vi "postiontesting.vi"() -> ()   [LabVIEW 2017]
uses:
  <vilib>/Simulation/Scripting/Companion Diagram/SimConfigNode/SimParams.ctl
  <vilib>/Simulation/Scripting/Companion Diagram/SimConfigNode/_simSolvers.ctl
  <vilib>/Simulation/Implementation/Shared/SIMSCR Execution Mode.ctl
  <vilib>/Simulation/Param Hierarchy/Typedefs/SIMPH Param Control Actions.ctl
  <vilib>/Simulation/Implementation/Shared/NILVSim_ParamChanged.vi
  <vilib>/Simulation/Implementation/Shared/NILVSIM_BeginStep.vi
  <vilib>/Simulation/Implementation/Shared/NILVSim_Manager.vi
  <vilib>/Utility/error.llb/Clear Errors.vi
  <vilib>/Simulation/Implementation/Shared/NILVSim_FinalizeModel.vi
  <vilib>/DAQmx/read.llb/DAQmx Read (Counter DBL 1Chan 1Samp).vi
  <vilib>/DAQmx/read.llb/DAQmx Read (Digital Bool 1Line 1Point).vi
  <vilib>/DAQmx/write.llb/DAQmx Write (Analog DBL 1Chan 1Samp).vi
  <vilib>/DAQmx/create/channels.llb/DAQmx Create Channel (AO-Voltage-Basic).vi
  <vilib>/DAQmx/create/channels.llb/DAQmx Create Channel (DI-Digital Input).vi
  <vilib>/DAQmx/create/channels.llb/DAQmx Create Channel (CI-Count Edges).vi
  <vilib>/Simulation/Implementation/Shared/SIM Unbundle Sim Info.vi
  <vilib>/Simulation/Implementation/Shared/NILVSim_Initialize.vi
  <vilib>/Simulation/Utility/Implementation/NILVSim Get Time and IsAcceptedStep.vi
  <vilib>/Simulation/Implementation/Shared/SIMSH Read Queue.vi
  <vilib>/Simulation/Implementation/Shared/NILVSim_GetModelError.vi
  <vilib>/Simulation/Implementation/Shared/SIM Bundle Sim Info.vi
  <vilib>/DAQmx/miscellaneous.llb/DAQmx Fill In Error Info.vi
  <vilib>/Simulation/Implementation/XNodeFramework/SimXNode/SimX.xnode
  <vilib>/Simulation/Model Libraries/PID/SIM PID (Parallel).vi
  <vilib>/Simulation/Model Libraries/PID/SIM PID.vi
  <vilib>/Simulation/Scripting/Companion Diagram/SimConfigNode/SimDog.xnode
  <vilib>/Simulation/Model Libraries/PID/SIM PID (Academic).vi
  <vilib>/Simulation/Implementation/Shared/NI_SIM_Implementation.lvlib
panel:
  in  "Draw rectangle":bool
  in  "Draw circle":bool
  out "In drawing mode":bool
  in  "Right-Down":bool
  in  "Left-Up":bool
  in  "Left-Down":bool
  in  "Right-Up":bool
  in  "right":bool
  in  "left":bool
  in  "motor 2":dbl(slide)=1.5 scale=-10.0..10.0
  in  "down":bool
  in  "up":bool
  in  "Length 2":dbl
  in  "Length 1":dbl
  in  "Motor 2 encoder":tag="Dev9/ao0"
  out "Pulses M2":dbl format="%.2f"
  in  "Motor 1 encoder":tag="Dev9/ao0"
  out "Pulses M1":dbl format="%.2f"
  out "Right":bool
  out "Bottom":bool
  out "Left":bool
  out "Top":bool
  in  "Switch 4/Line 3":tag
  in  "Switch 3/Line 2":tag
  in  "Switch 2/Line 1":tag
  in  "Switch 1/Line 0":tag
  in  "Motor stop":bool
  in  "Motor 1":tag="Dev9/ao0"
  in  "max Voltage":dbl
  in  "Min Voltage":dbl
  in  "Motor 2":tag="Dev9/ao0"
  in  "motor 1":dbl(slide)=1.5 scale=-10.0..10.0
  in  "stop":bool
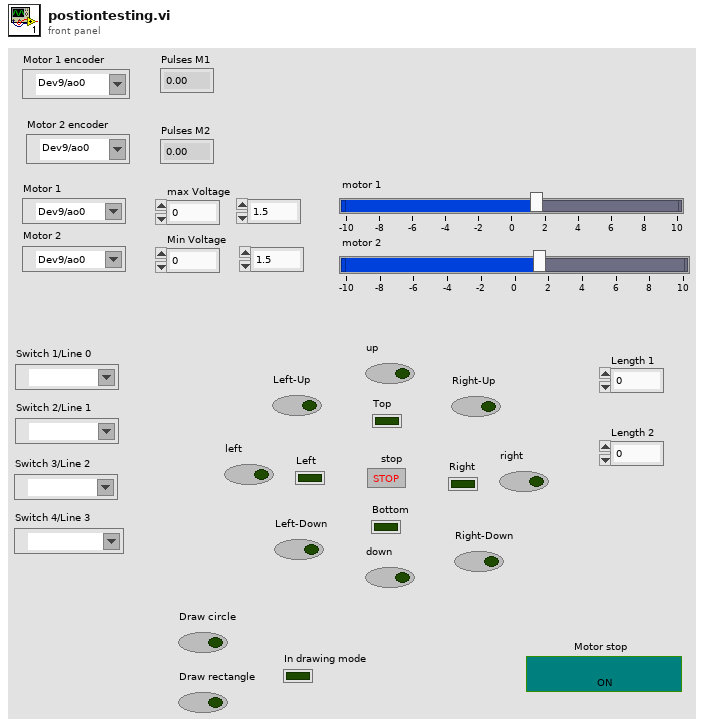
[diagram p1: front panel]
types:
  T1 = enum16{"Simulate to Completion", "Single Time-Step Simulation (Fixed Step Only)"}
  T2 = typedef "SIMSCR Execution Mode.ctl" = enum16{"Simulate to Completion", "Single Time-Step Simulation (Fixed Step Only)"}
  T3 = typedef "SIMPH Param Control Actions.ctl" = enum16{"get params", "set params"}
  T4 = cluster{"SIMSH Sim Time":dbl, "SIM PID Derivative Gain.vi":cluster{"output":dbl}, "SIM PID Derivative Gain.vi - SIMSH":cluster{"SIMSH Sim Time":dbl, "t 3":dbl, "Select 2":cluster{"s? t:f":dbl}, "Equal?":cluster{"x = y?":bool}, "Or":cluster{"x .or. y?":bool}, "Equal To 0?":cluster{"x = 0?":bool}}, "High Frequency [s] (Tf)":dbl, "Gain":cluster{"output":dbl}, "Summation":cluster{"Result":dbl}, "Integral Gain - series.vi":cluster{"output":dbl}, "Integral Gain - series.vi - SIMSH":cluster{"SIMSH Sim Time":dbl, "Select 2":cluster{"s? t:f":dbl}, "integral in gain?":bool, "Integrator":cluster{"output y(t)":dbl}, "Gain 2":cluster{"output":dbl}, "Select":cluster{"s? t:f":dbl}, "Equal To 0?":cluster{"x = 0?":bool}, "Reciprocal":cluster{"1/x":dbl}}}
  T5 = typedef "SimParams.ctl" = cluster{"Initial Time (s)":dbl, "Final Time (s)":dbl, "Step Size (s)":dbl, "ODE Solver":T6, "Minimum Step Size (s)":dbl, "Maximum Step Size (s)":dbl, "Relative Tolerance":dbl, "Absolute Tolerance":dbl, "Software Timing":bool, "Initial Step Size (s)":dbl, "Automatic Fixed Step Size?":bool, "Automatic Discrete Step Size?":bool, "Discrete Step Size (s)":dbl, "Calculate using Time Step":bool, "Solver Wired?":bool, "Prev.Frm.Expected End":u64, "Prev.Frm.Actual End":u64, "Prev.Frm.Finished Late?":bool, "Prev.Iter.Expected End":u64, "Prev.Iter.Actual End":u64, "Prev.Iter.Finished Late?":bool, "Expected Iteration Start":u64, "Actual Iteration Start":u64, "Expected Frame Start":u64, "Actual Frame Start":u64, "Source Name":string, "Name":string, "Period":i64, "Deadline":i64, "Offset":i64, "Start":i64, "Priority":i32, "Timeout":i32, "Processor":i32, "Mode":enum32{"No Change", "Process missed periods, maintain original phase", "Discard missed periods, maintain original phase", "Process missed periods, ignore original phase", "Discard missed periods, ignore original phase"}, "Wakeup reason":enum32{"Normal", "Aborted", "Asynchronous wakeup", "Timing source error", "Timed loop error", "Timeout"}, "Error":errorcluster, "Source Type":string, "Secondary Source Type":string, "Global End Time":u64, "Global Start Time":u64, "Full Solver Reset":bool, "Execution Mode":T2, "Nan/Inf Check":bool, "Custom Solver Library":string, "Solver Is Variable":bool, "custom solver name":string, "Signal Collection Decimation":u32}
  T6 = typedef "_simSolvers.ctl" = enum16{"Runge-Kutta 1 (Euler)", "Runge-Kutta 2", "Runge-Kutta 3", "Runge-Kutta 4", "Runge-Kutta 23 (variable)", "Runge-Kutta 45 (variable)", "BDF (variable)", "Adams-Moulton (variable)", "Rosenbrock (variable)", "Discrete States Only", "SDIRK 4 (variable)", "Radau 5 (variable)", "Radau 9 (variable)", "Radau 13 (variable)", "Radau [Variable Order] (variable)", "Gear's Method (variable)", "Linearizer", "State Query", "Trim Eval", "Custom Solver"}
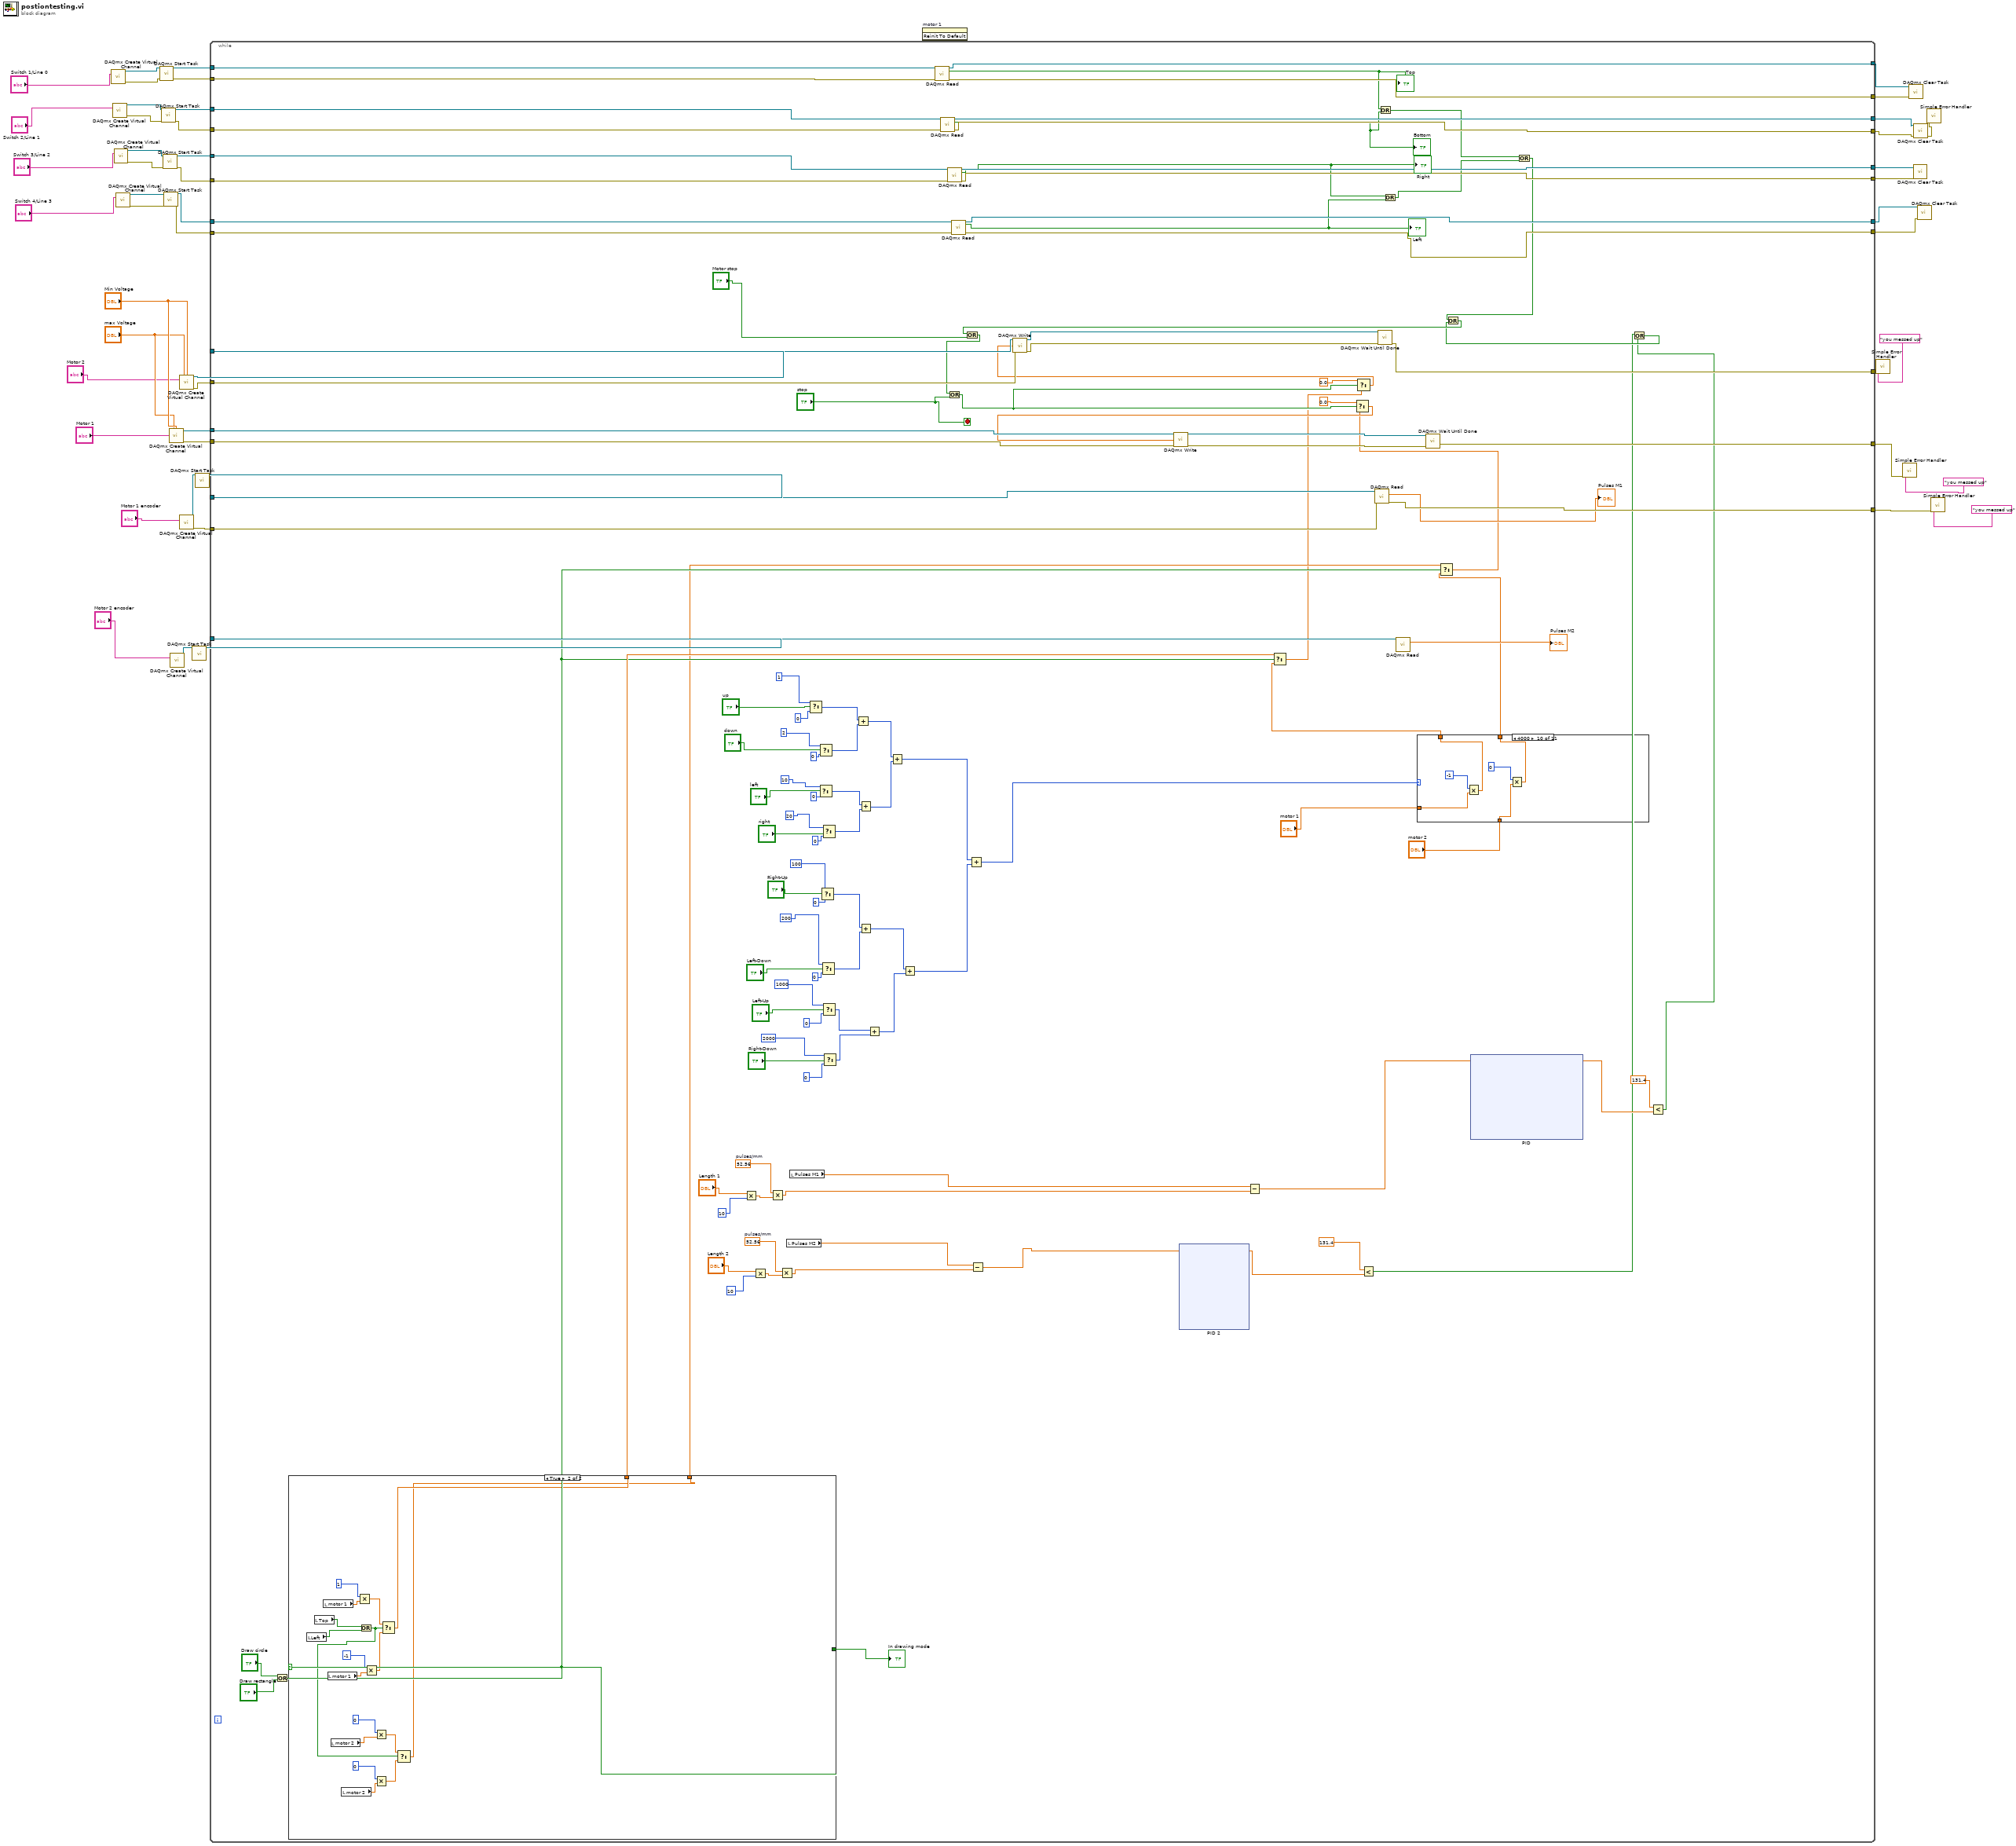
[diagram p0: block diagram]
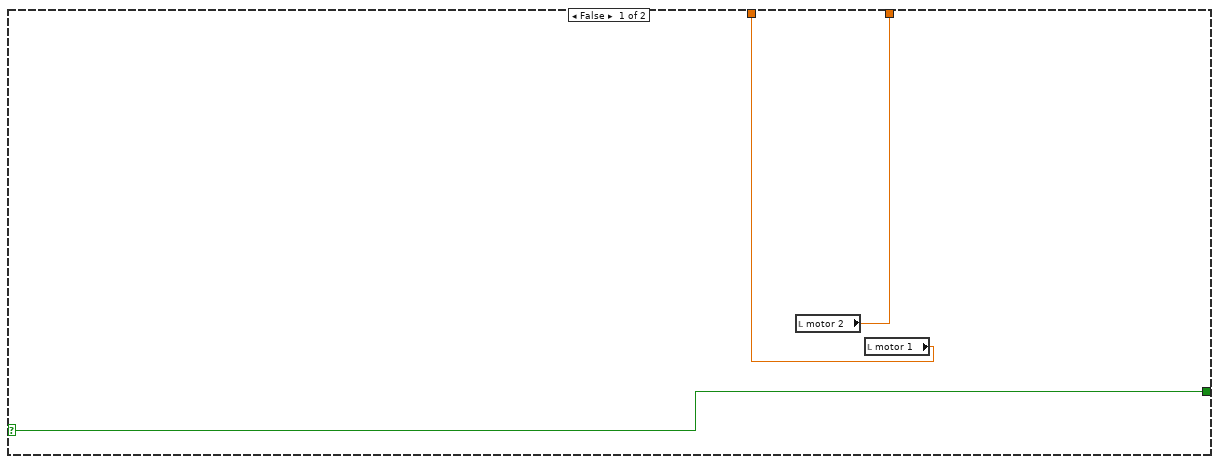
[diagram p2: hidden frame]
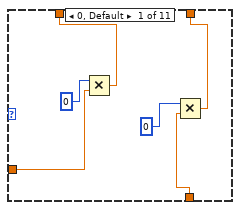
[diagram p3: hidden frame]
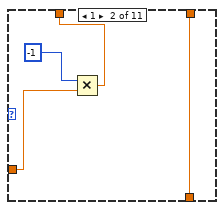
[diagram p4: hidden frame]
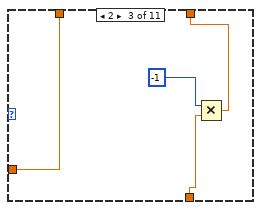
[diagram p5: hidden frame]
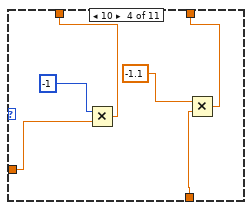
[diagram p6: hidden frame]
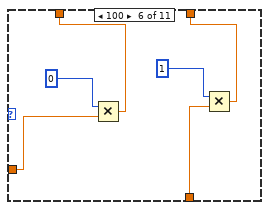
[diagram p8: hidden frame]
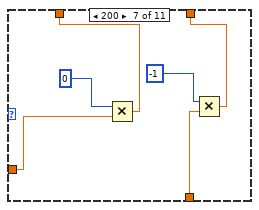
[diagram p9: hidden frame]
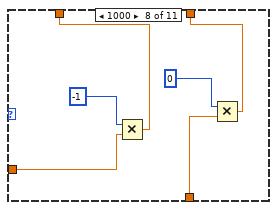
[diagram p10: hidden frame]
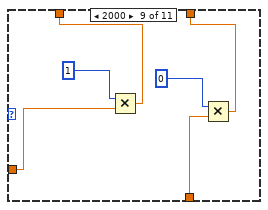
[diagram p11: hidden frame]
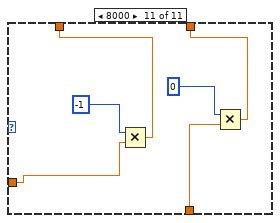
[diagram p12: hidden frame]
diagram:
  n1 = call-poly <vilib>:"DAQmx Create Virtual Channel.vi"("lines"="Switch 1/Line 0") -> ("task out"=w36:refnum<k21>, "error out"=w32:errorcluster)  [unwired: 13 in]
  n2 = call-poly <vilib>:"DAQmx Create Virtual Channel.vi"("lines"="Switch 2/Line 1") -> ("task out"=w35:refnum<k21>, "error out"=w31:errorcluster)  [unwired: 13 in]
  n3 = call-poly <vilib>:"DAQmx Create Virtual Channel.vi"("lines"="Switch 3/Line 2") -> ("task out"=w34:refnum<k21>, "error out"=w30:errorcluster)  [unwired: 13 in]
  n4 = call-poly <vilib>:"DAQmx Create Virtual Channel.vi"("lines"="Switch 4/Line 3") -> ("task out"=w33:refnum<k21>, "error out"=w29:errorcluster)  [unwired: 13 in]
  n5 = call <vilib>:"DAQmx Start Task.vi"("task/channels in"=w36, "error in"=w32) -> ("task out"=w28:refnum<k21>, "error out"=w26:errorcluster)  [unwired: 12 in]
  n6 = call <vilib>:"DAQmx Start Task.vi"("task/channels in"=w35, "error in"=w31) -> ("task out"=w24:refnum<k21>, "error out"=w21:errorcluster)  [unwired: 12 in]
  n7 = call <vilib>:"DAQmx Start Task.vi"("task/channels in"=w34, "error in"=w30) -> ("task out"=w23:refnum<k21>, "error out"=w20:errorcluster)  [unwired: 12 in]
  n8 = call <vilib>:"DAQmx Start Task.vi"("task/channels in"=w33, "error in"=w29) -> ("task out"=w22:refnum<k21>, "error out"=w19:errorcluster)  [unwired: 12 in]
  n9 = call-poly <vilib>:"DAQmx Create Virtual Channel.vi"("maximum value"="max Voltage", "minimum value"="Min Voltage", "physical channels"="Motor 1") -> ("task out"=w46:refnum<k21>, "error out"=w42:errorcluster)  [unwired: 11 in]
  n10 = call-poly <vilib>:"DAQmx Create Virtual Channel.vi"("counter"="Motor 2 encoder") -> ("task out"=w4:refnum<k21>)  [unwired: 13 in, 1 out]
  n11 = call-poly <vilib>:"DAQmx Create Virtual Channel.vi"("maximum value"="max Voltage", "minimum value"="Min Voltage", "physical channels"="Motor 2") -> ("task out"=w49:refnum<k21>, "error out"=w41:errorcluster)  [unwired: 11 in]
  n12 = call-poly <vilib>:"DAQmx Create Virtual Channel.vi"("counter"="Motor 1 encoder") -> ("task out"=w6:refnum<k21>, "error out"=w7:errorcluster)  [unwired: 13 in]
  n13 = call <vilib>:"DAQmx Start Task.vi"("task/channels in"=w4) -> ("task out"=w3:refnum<k21>)  [unwired: 13 in, 1 out]
  n14 = call <vilib>:"DAQmx Start Task.vi"("task/channels in"=w6) -> ("task out"=w5:refnum<k21>)  [unwired: 13 in, 1 out]
  n15 = while {
    tunnel: w49 -> [w170]
    tunnel: [w167] -> w48
    tunnel: w46 -> [w164]
    tunnel: [w163] -> w45
    tunnel: w42 -> [w161]
    tunnel: w41 -> [w160]
    tunnel: w28 -> [w154]
    tunnel: [w153] -> w27
    tunnel: w26 -> [w152]
    tunnel: [w151] -> w25
    tunnel: w24 -> [w150]
    tunnel: w23 -> [w149]
    tunnel: w22 -> [w148]
    tunnel: w21 -> [w147]
    tunnel: w20 -> [w146]
    tunnel: w19 -> [w145]
    tunnel: [w144] -> w18
    tunnel: [w143] -> w17
    tunnel: [w142] -> w16
    tunnel: [w141] -> w15
    tunnel: [w140] -> w14
    tunnel: [w139] -> w13
    tunnel: [w138] -> w10
    tunnel: w5 -> [w137]
    tunnel: w7 -> [w136]
    tunnel: w3 -> [w127]
    stop <- "stop" stop-if-true
    w117 = 52.56  # pulses/mm
    w122 = 52.56  # pulses/mm
    n16 = Or(x="Draw circle", y="Draw rectangle") -> (x .or. y?=w56:bool)
    n17 = case shown="True" w56 {
      selector: w56 -> [w173 w191]
      tunnel: [w173 w191] -> w60
      tunnel: [w172 w176] -> w57
      tunnel: [w171 w175] -> w55
      frame False {
        n18 = local read "motor 2"() -> (w171:dbl)
        n19 = local read "motor 1"() -> (w172:dbl)
      }
      frame True {
        n20 = local read "Left"() -> (w174:bool)
        n21 = local read "Top"() -> (w190:bool)
        n22 = local read "motor 1"() -> (w187:dbl)
        n23 = local read "motor 1"() -> (w181:dbl)
        n24 = local read "motor 2"() -> (w185:dbl)
        n25 = local read "motor 2"() -> (w178:dbl)
        n26 = Multiply(x=1, y=w187) -> (x*y=w186:dbl)
        n27 = Or(x=w190, y=w174) -> (x .or. y?=w183:bool)
        n28 = Multiply(x=-1, y=w181) -> (x*y=w180:dbl)
        n29 = Multiply(x=0, y=w185) -> (x*y=w184:dbl)
        n30 = Multiply(x=0, y=w178) -> (x*y=w177:dbl)
        n31 = Select(t=w186, s=w183, f=w180) -> (s? t:f=w176:dbl)
        n32 = Select(t=w184, s=w183, f=w177) -> (s? t:f=w175:dbl)
      }
    }
    "In drawing mode" <- w60
    n33 = Multiply(x="Length 1", y=10) -> (x*y=w121:dbl)
    n34 = Multiply(x="Length 2", y=10) -> (x*y=w120:dbl)
    n35 = Multiply(x=w122, y=w121) -> (x*y=w110:dbl)
    n36 = Multiply(x=w117, y=w120) -> (x*y=w104:dbl)
    n37 = local read "Pulses M2"() -> (w105:dbl)
    n38 = local read "Pulses M1"() -> (w111:dbl)
    n39 = Select(t=1, s="up", f=0) -> (s? t:f=w84:i32)
    n40 = Select(t=10, s="left", f=0) -> (s? t:f=w82:i32)
    n41 = Select(t=2, s="down", f=0) -> (s? t:f=w83:i32)
    n42 = Select(t=100, s="Right-Up", f=0) -> (s? t:f=w80:i32)
    n43 = Select(t=200, s="Left-Down", f=0) -> (s? t:f=w79:i32)
    n44 = Select(t=20, s="right", f=0) -> (s? t:f=w81:i32)
    n45 = Select(t=1000, s="Left-Up", f=0) -> (s? t:f=w78:i32)
    n46 = Select(t=2000, s="Right-Down", f=0) -> (s? t:f=w64:i32)
    n47 = Add(x=w84, y=w83) -> (x+y=w77:i32)
    n48 = Add(x=w82, y=w81) -> (x+y=w76:i32)
    n49 = Add(x=w80, y=w79) -> (x+y=w75:i32)
    n50 = Add(x=w78, y=w64) -> (x+y=w63:i32)
    n51 = Add(x=w77, y=w76) -> (x+y=w74:i32)
    n52 = Add(x=w75, y=w63) -> (x+y=w62:i32)
    n53 = call-poly <vilib>:"DAQmx Read.vi"("task/channels in"=w154, "error in"=w152) -> ("task out"=w153:refnum<k21>, "data"=w135:bool, "error out"=w151:errorcluster)  [unwired: 11 in]
    "Top" <- w135
    n54 = call-poly <vilib>:"DAQmx Read.vi"("task/channels in"=w150, "error in"=w147) -> ("task out"=w144:refnum<k21>, "data"=w134:bool, "error out"=w141:errorcluster)  [unwired: 11 in]
    "Bottom" <- w134
    n55 = call-poly <vilib>:"DAQmx Read.vi"("task/channels in"=w149, "error in"=w146) -> ("task out"=w143:refnum<k21>, "data"=w132:bool, "error out"=w140:errorcluster)  [unwired: 11 in]
    "Right" <- w132
    n56 = call-poly <vilib>:"DAQmx Read.vi"("task/channels in"=w148, "error in"=w145) -> ("task out"=w142:refnum<k21>, "data"=w131:bool, "error out"=w139:errorcluster)  [unwired: 11 in]
    "Left" <- w131
    n57 = Add(x=w74, y=w62) -> (x+y=w61:i32)
    n58 = Subtract(x=w105, y=w104) -> (x-y=w103:dbl)
    n59 = xnode "PID 2"("Error"=w103) -> ("Output"=w101:dbl)  [unwired: 2 in, 11 out]
    n60 = Subtract(x=w111, y=w110) -> (x-y=w109:dbl)
    n61 = Less?(x=131.4, y=w101) -> (x < y?=w100:bool)
    n62 = call-poly <vilib>:"DAQmx Read.vi"("task/channels in"=w137, "error in"=w136) -> ("data"=→"Pulses M1":dbl, "error out"=w138:errorcluster)  [unwired: 11 in, 1 out]
    n63 = Or(x=w135, y=w134) -> (x .or. y?=w133:bool)
    n64 = Or(x=w132, y=w131) -> (x .or. y?=w130:bool)
    n65 = call-poly <vilib>:"DAQmx Read.vi"("task/channels in"=w127) -> ("data"=→"Pulses M2":dbl)  [unwired: 12 in, 2 out]
    n66 = case shown="4000" w61 {
      tunnel: "motor 1" -> [w690 w693 w696 w703 w707 w711 w717 w723 w729 w734 w741]
      tunnel: "motor 2" -> [w687 w695 w698 w701 w706 w709 w715 w721 w727 w735 w740]
      tunnel: [w686 w695 w697 w700 w706 w708 w714 w720 w726 w732 w739] -> w52
      tunnel: [w689 w692 w696 w702 w707 w710 w716 w722 w728 w733 w738] -> w54
      frame 0, Default {
        n67 = Multiply(x=0, y=w690) -> (x*y=w689:dbl)
        n68 = Multiply(x=0, y=w687) -> (x*y=w686:dbl)
      }
      frame 1 {
        n69 = Multiply(x=-1, y=w693) -> (x*y=w692:dbl)
      }
      frame 2 {
        n70 = Multiply(x=-1, y=w698) -> (x*y=w697:dbl)
      }
      frame 10 {
        n71 = Multiply(x=-1, y=w703) -> (x*y=w702:dbl)
        n72 = Multiply(x=-1.1, y=w701) -> (x*y=w700:dbl)
      }
      frame 20 {
      }
      frame 100 {
        n73 = Multiply(x=0, y=w711) -> (x*y=w710:dbl)
        n74 = Multiply(x=1, y=w709) -> (x*y=w708:dbl)
      }
      frame 200 {
        n75 = Multiply(x=0, y=w717) -> (x*y=w716:dbl)
        n76 = Multiply(x=-1, y=w715) -> (x*y=w714:dbl)
      }
      frame 1000 {
        n77 = Multiply(x=-1, y=w723) -> (x*y=w722:dbl)
        n78 = Multiply(x=0, y=w721) -> (x*y=w720:dbl)
      }
      frame 2000 {
        n79 = Multiply(x=1, y=w729) -> (x*y=w728:dbl)
        n80 = Multiply(x=0, y=w727) -> (x*y=w726:dbl)
      }
      frame 4000 {
        n81 = Multiply(x=-1, y=w734) -> (x*y=w733:dbl)
        n82 = Multiply(x=0, y=w735) -> (x*y=w732:dbl)
      }
      frame 8000 {
        n83 = Multiply(x=-1, y=w741) -> (x*y=w738:dbl)
        n84 = Multiply(x=0, y=w740) -> (x*y=w739:dbl)
      }
    }
    n85 = Select(t=w57, s=w56, f=w54) -> (s? t:f=w53:dbl)
    n86 = Select(t=w55, s=w56, f=w52) -> (s? t:f=w51:dbl)
    n87 = xnode "PID"("Error"=w109) -> ("Output"=w108:dbl)  [unwired: 2 in, 11 out]
    n88 = Or(x=w133, y=w130) -> (x .or. y?=w126:bool)
    n89 = Less?(x=131.4, y=w108) -> (x < y?=w106:bool)
    n90 = Or(x=w100, y=w106) -> (x .or. y?=w116:bool)
    n91 = Or(x=w126, y=w116) -> (x .or. y?=w125:bool)
    n92 = Or(x=w125, y="Motor stop") -> (x .or. y?=w129:bool)
    n93 = Or(x=w129, y="stop") -> (x .or. y?=w158:bool)
    n94 = Select(t=0.0, s=w158, f=w51) -> (s? t:f=w155:dbl)
    n95 = call-poly <vilib>:"DAQmx Write.vi"("task/channels in"=w164, "data"=w155, "error in"=w161) -> ("task out"=w165:refnum<k21>, "error out"=w166:errorcluster)  [unwired: 10 in, 1 out]
    n96 = Select(t=0.0 ("s? t:f"), s=w158, f=w53) -> (s? t:f=w156:dbl)
    n97 = call-poly <vilib>:"DAQmx Write.vi"("task/channels in"=w170, "data"=w156, "error in"=w160) -> ("task out"=w169:refnum<k21>, "error out"=w168:errorcluster)  [unwired: 10 in, 1 out]
    n98 = call <vilib>:"DAQmx Wait Until Done.vi"("task/channels in"=w169, "error in"=w168) -> ("error out"=w167:errorcluster)  [unwired: 12 in, 1 out]
    n99 = call <vilib>:"DAQmx Wait Until Done.vi"("task/channels in"=w165, "error in"=w166) -> ("error out"=w163:errorcluster)  [unwired: 12 in, 1 out]
  }
  n100 = invoke on="motor 1" class="Slide (strict)" method="Reinit To Default"() -> ()  [unwired: 3 in, 3 out]
  n101 = call <vilib>:"Simple Error Handler.vi"("error source (\" \")"="you messed up" ("error source (\" \")"), "error in (no error)"=w48) -> ()  [unwired: 3 in, 5 out]
  n102 = call <vilib>:"Simple Error Handler.vi"("error source (\" \")"="you messed up" ("error source (\" \")"), "error in (no error)"=w45) -> ()  [unwired: 3 in, 5 out]
  n103 = call <vilib>:"DAQmx Clear Task.vi"("task in"=w27, "error in"=w25) -> ()  [unwired: 13 in, 1 out]
  n104 = call <vilib>:"DAQmx Clear Task.vi"("task in"=w17, "error in"=w14) -> ()  [unwired: 13 in, 1 out]
  n105 = call <vilib>:"DAQmx Clear Task.vi"("task in"=w18, "error in"=w15) -> ("error out"=w12:errorcluster)  [unwired: 13 in]
  n106 = call <vilib>:"DAQmx Clear Task.vi"("task in"=w16, "error in"=w13) -> ()  [unwired: 13 in, 1 out]
  n107 = call <vilib>:"Simple Error Handler.vi"("error in (no error)"=w12) -> ()  [unwired: 4 in, 5 out]
  n108 = call <vilib>:"Simple Error Handler.vi"("error source (\" \")"="you messed up" ("error source (\" \")"), "error in (no error)"=w10) -> ()  [unwired: 3 in, 5 out]
